vi "fox.vi"() -> ()   [LabVIEW 2015]
panel:
  in  "stop 2":bool
  out "Numeric":i32
  out "R":bool
  out "Y":bool
  out "G":bool
  in  "stop":bool
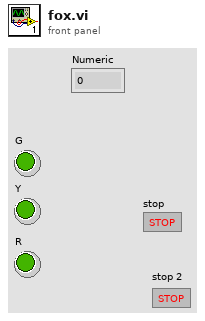
[diagram p1: front panel]
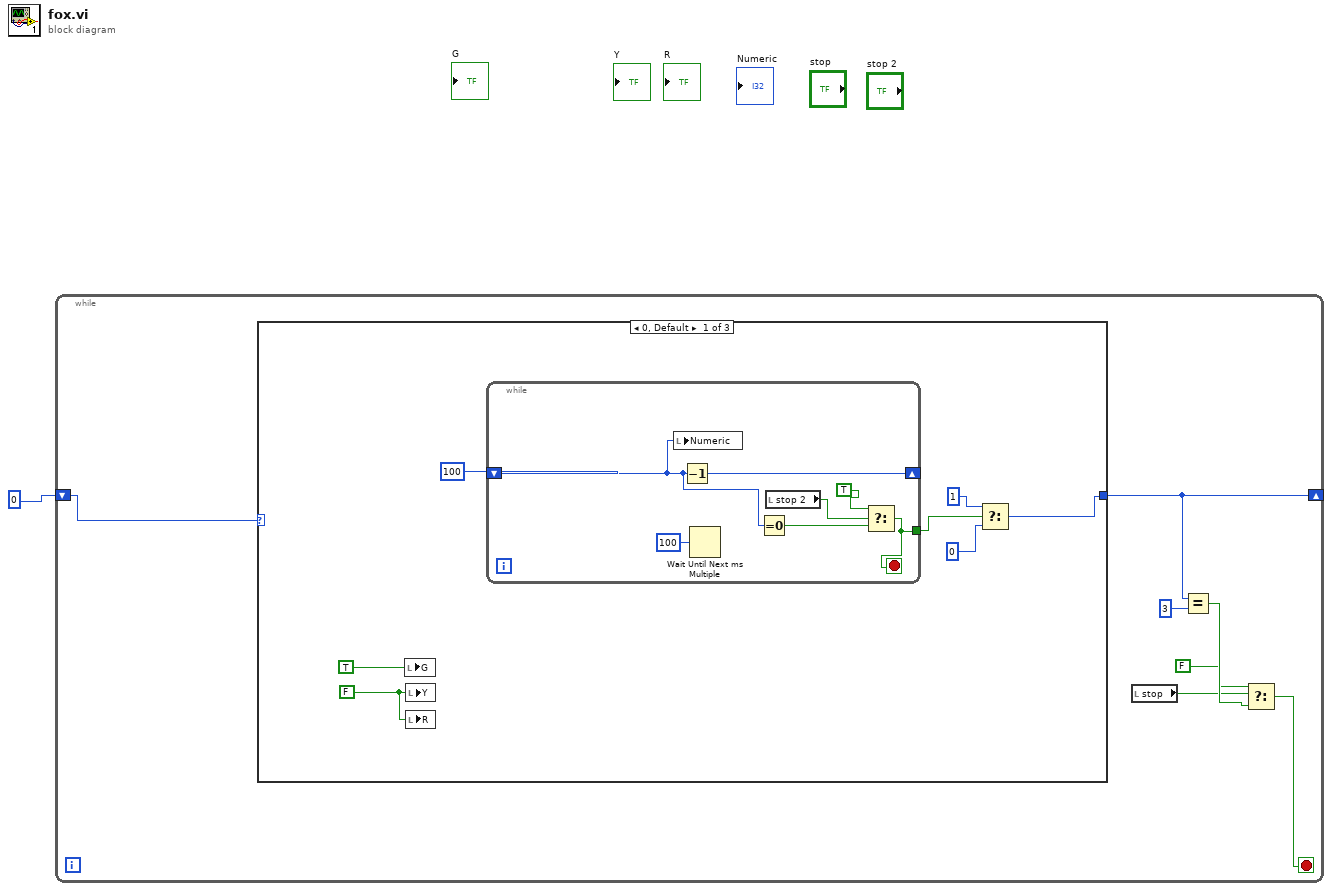
[diagram p0: block diagram]
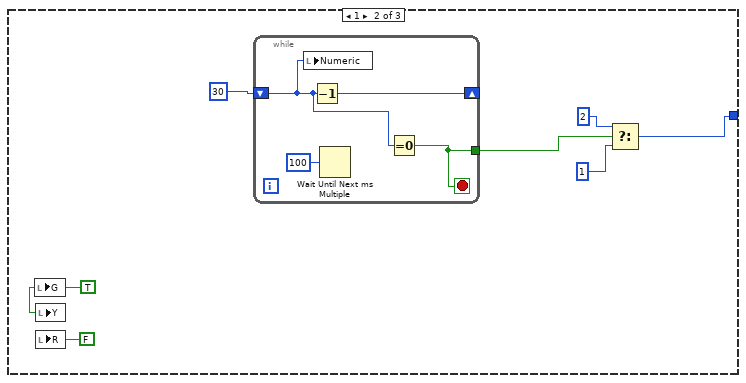
[diagram p2: hidden frame]
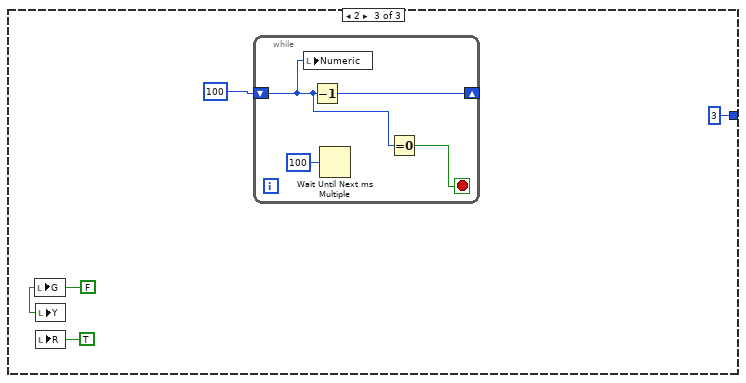
[diagram p3: hidden frame]
diagram:
  n1 = while {
    shift-right: [w7] -> _
    shift-left: 0 -> [w8]
    stop <- w2 stop-if-true
    n2 = case shown="0, Default" w8 {
      tunnel: [w9 w25 u32 3 ("millisecond multiple")] -> w7
      frame 0, Default {
        w14 = FALSE ("G")
        n3 = local write "G"(TRUE ("G")) -> ()
        n4 = local write "Y"(w14) -> ()
        n5 = local write "R"(w14) -> ()
        n6 = while {
          shift-right: [w22] -> _
          shift-left: u32 100 ("millisecond multiple") -> [w16]
          tunnel: [w17] -> w12
          stop <- w17 stop-if-true
          n7 = local write "Numeric"(w16) -> ()
          n8 = Decrement(x=w16) -> (x-1=w22:u32)
          n9 = Wait Until Next ms Multiple(millisecond multiple=u32 100) -> ()  [unwired: 1 out]
          n10 = Equal To 0?(x=w16) -> (x = 0?=w18:bool)
          n11 = local read "stop 2"() -> (w20:bool)
          n12 = Select(t=TRUE ("G"), s=w20, f=w18) -> (s? t:f=w17:bool)
        }
        n13 = Select(t=u32 1 ("millisecond multiple"), s=w12, f=u32 0 ("millisecond multiple")) -> (s? t:f=w9:u32)
      }
      frame 1 {
        w23 = TRUE ("G")
        n14 = local write "G"(w23) -> ()
        n15 = local write "Y"(w23) -> ()
        n16 = local write "R"(FALSE ("G")) -> ()
        n17 = while {
          shift-right: [w33] -> _
          shift-left: u32 30 ("millisecond multiple") -> [w30]
          tunnel: [w31] -> w28
          stop <- w31 stop-if-true
          n18 = local write "Numeric"(w30) -> ()
          n19 = Decrement(x=w30) -> (x-1=w33:u32)
          n20 = Wait Until Next ms Multiple(millisecond multiple=u32 100) -> ()  [unwired: 1 out]
          n21 = Equal To 0?(x=w30) -> (x = 0?=w31:bool)
        }
        n22 = Select(t=u32 2 ("millisecond multiple"), s=w28, f=u32 1 ("millisecond multiple")) -> (s? t:f=w25:u32)
      }
      frame 2 {
        w35 = FALSE ("G")
        n23 = local write "G"(w35) -> ()
        n24 = local write "Y"(w35) -> ()
        n25 = local write "R"(TRUE ("G")) -> ()
        n26 = while {
          shift-right: [w41] -> _
          shift-left: u32 100 ("millisecond multiple") -> [w38]
          stop <- w39 stop-if-true
          n27 = local write "Numeric"(w38) -> ()
          n28 = Decrement(x=w38) -> (x-1=w41:u32)
          n29 = Wait Until Next ms Multiple(millisecond multiple=u32 100) -> ()  [unwired: 1 out]
          n30 = Equal To 0?(x=w38) -> (x = 0?=w39:bool)
        }
      }
    }
    n31 = local read "stop"() -> (w4:bool)
    n32 = Equal?(x=w7, y=u32 3) -> (x = y?=w5:bool)
    n33 = Select(t=FALSE, s=w4, f=w5) -> (s? t:f=w2:bool)
  }
